vi "Change Theme.vi"(8 "error in":errorcluster, 11 "VI Refnum":refnum<vi>) -> (0 "error out":errorcluster)   [LabVIEW 2021]
doc: "Show this VI and let user define a new path/theme to apply to the VI.\n\n->Will be invoked with Quick Drop as a way to easily change the theme quickly during edit mode\n\n<b>Code Developed By:</b>\nTechnology Service Corporation\nwww.tsc.com/atcs\n\nDeveloper:\nDaniel Coons"
uses:
  Material Theme/Material Theme.lvclass
  user32.dll
panel:
  out "Name of VI":string
  in  "Theme":u16(ring) items=["Light", "Light Medium Contrast", "Light High Contrast", "Dark", "Dark Medium Contrast", "Dark High Contrast"]
  in  "done":bool
  out "header":bool
  in  "Path to theme file":path
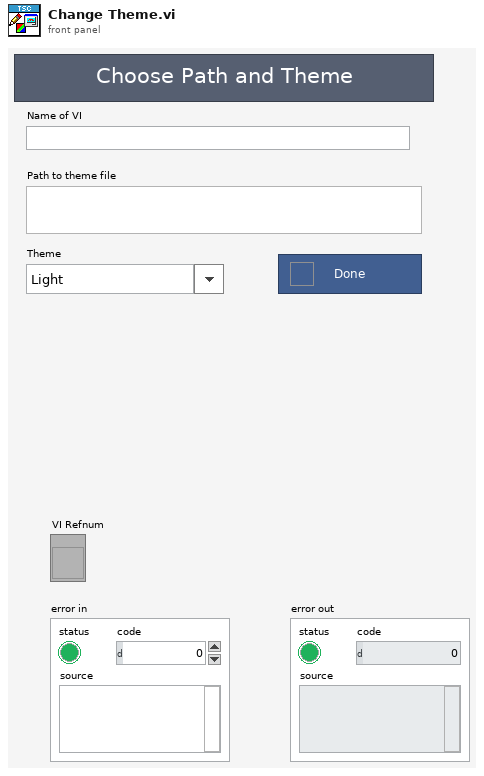
[diagram p1: front panel]
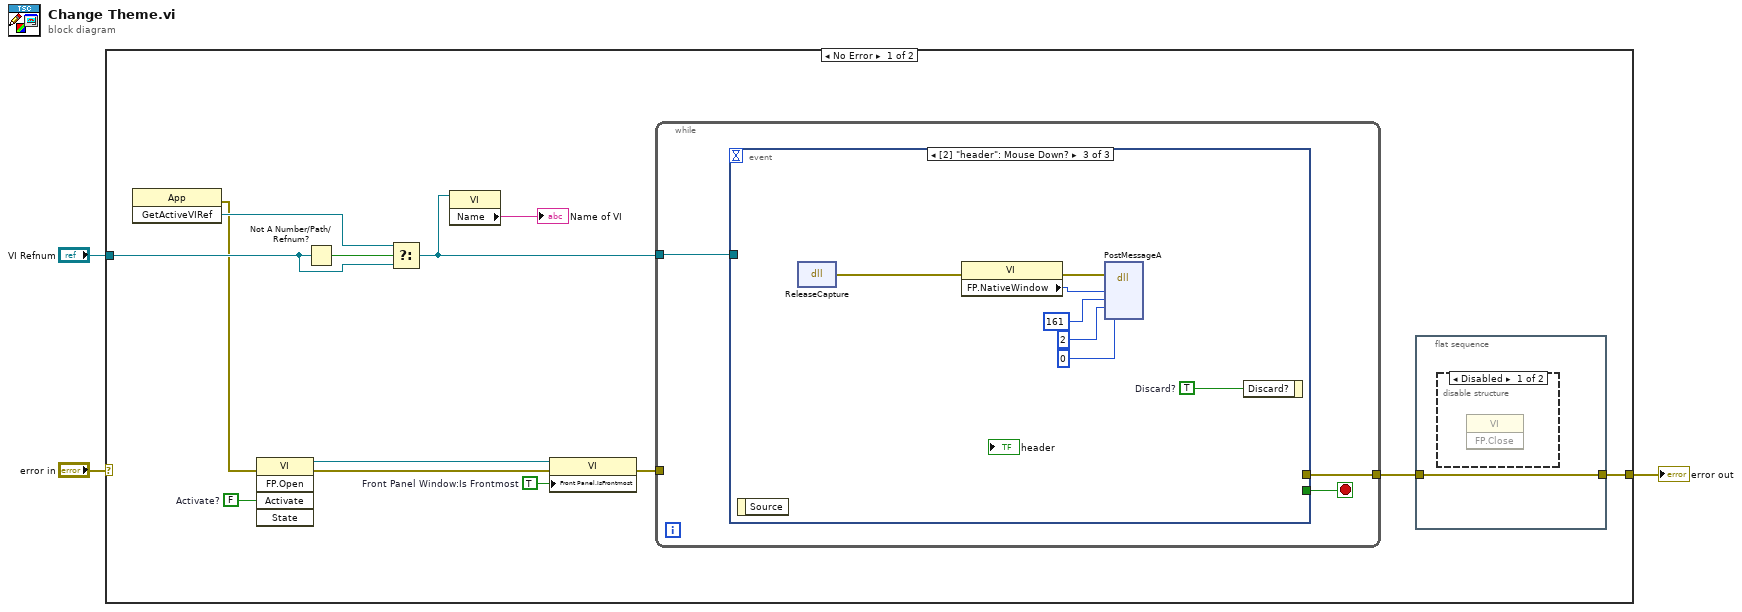
[diagram p0: block diagram]
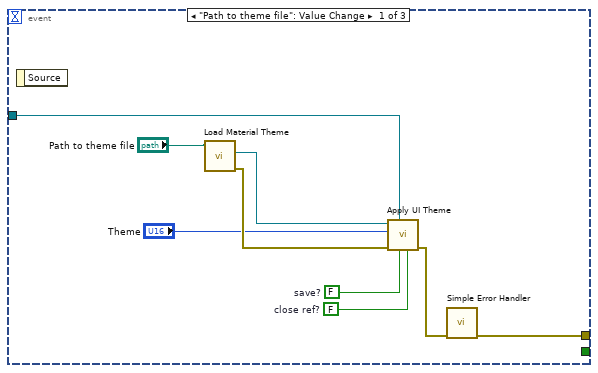
[diagram p3: hidden frame]
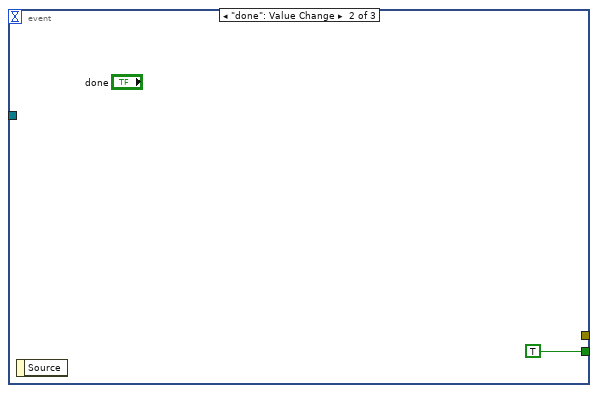
[diagram p4: hidden frame]
diagram:
  n1 = case shown="No Error" "error in" {
    selector: "error in" -> [_ w38]
    tunnel: "VI Refnum" -> [w7 _]
    tunnel: [w13 w38] -> w2
    frame No Error {
      w10 = TRUE  # Front Panel Window:Is Frontmost
      w15 = FALSE  # Activate?
      n2 = invoke class="App" method="GetActiveVIRef"() -> (error out=w4:errorcluster, "GetActiveVIRef"=w8:refnum<vi>)  [unwired: 3 in, 1 out]
      n3 = invoke class="VI" method="FP.Open"(error in=w4, "Activate"=w15) -> (reference out=w11:refnum<vi>, error out=w16:errorcluster)  [unwired: 3 in, 3 out]
      n4 = Not A Number/Path/Refnum?(number/path/refnum=w7) -> (NaN/Path/Refnum?=w9:bool)
      n5 = Select(t=w8, s=w9, f=w7) -> (s? t:f=w6:refnum<vi>)
      n6 = property class="VI"(reference=w6) -> ("Name"=→"Name of VI":string)  [unwired: 1 in, 2 out]
      n7 = property class="VI"(reference=w11, error in=w16, "Front Panel.IsFrontmost"=w10) -> (error out=w12:errorcluster)  [unwired: 1 out]
      n8 = while {
        tunnel: w6 -> [w20]
        tunnel: w12 -> [_]
        tunnel: [w19] -> w14
        stop <- w18 stop-if-true
        n9 = event shown="[2] \"header\": Mouse Down?" {
          selector: _ -> [_ _ _]
          dyn-events: _ -> [_ _ _]
          timeout: _ -> [_ _ _]
          tunnel: w20 -> [w27 _ _]
          tunnel: [w24 _ _] -> w19
          tunnel: [_ TRUE _] -> w18
          event "Path to theme file": Value Change {
            w22 = FALSE  # save?
            w23 = FALSE  # close ref?
            n10 = event-data() -> ()  [unwired: 1 in, 1 out]
            n11 = call "Load Material Theme.vi"("file path (use dialog)"="Path to theme file") -> ("error out"=w26:errorcluster, "Theme"=w28:refnum<class "Material Theme.lvclass">)  [unwired: 9 in]
            n12 = call "Apply UI Theme.vi"("close ref?"=w23, "save?"=w22, "VI Refnum"=w27, "error in (no error)"=w26, "Theme"="Theme", "Material Theme in"=w28) -> ("error out"=w25:errorcluster)  [unwired: 4 in, 1 out]
            n13 = call <vilib>:"Simple Error Handler.vi"("error in (no error)"=w25) -> ("error out"=w24:errorcluster)  [unwired: 4 in, 4 out]
          }
          event "done": Value Change {
            n14 = event-data() -> ()  [unwired: 1 in, 1 out]
          }
          event "header": Mouse Down? {
            w37 = TRUE  # Discard?
            n15 = event-data() -> ()  [unwired: 1 in, 1 out]
            n16 = dll-call lib="user32.dll" fn="ReleaseCapture"() -> (error out=w33:errorcluster)  [unwired: 4 in, 1 out]
            n17 = property class="VI"(error in=w33) -> (error out=w32:errorcluster, "FP.NativeWindow"=w31:u64)  [unwired: 1 in, 1 out]
            n18 = dll-call lib="user32.dll" fn="PostMessageA"(error in=w32, "hWnd"=w31, "Msg"=161, "wParam"=2, "lParam"=0) -> ()  [unwired: 7 in, 2 out]
            n19 = event-data("Discard?"=w37) -> ()  [unwired: 1 in, 1 out]
          }
        }
      }
      n20 = flat-sequence {
        tunnel: w14 -> [w17]
        tunnel: [w17] -> w13
        frame #0 {
          n21 = disable-structure shown="Disabled" {
            frame Disabled {
              n22 = invoke class="VI" method="FP.Close"() -> ()  [unwired: 3 in, 3 out]
            }
            frame Enabled {
            }
          }
        }
      }
    }
    frame Error {
    }
  }
  "error out" <- w2
